vi "SVD demo.vi"(6 "number of points":i32(slide)=67 scale=0.0..600.0, 7 "gamma":dbl(slide) scale=-180.0..180.0, 8 "beta":dbl(slide) scale=-180.0..180.0, 9 "alpha":dbl(slide) scale=-180.0..180.0, 10 "length 2":dbl(slide)=5.0 scale=0.0..10.0, 11 "length 1":dbl(slide)=10.0 scale=0.0..10.0) -> ()   [LabVIEW 2009]
uses:
  <vilib>/Math Plots/3D Math Plots/3D Scatter/3D Scatter XCtrl/3D Scatter.xctl
  <vilib>/Math Plots/3D Math Plots/3D Scatter/3D Scatter Datatype/Public/Plot Helper (Vector).vi
  <vilib>/Analysis/Matrix/Numeric/Conversions/Matrix To Array - RM.vi
  <vilib>/Analysis/baseanly.llb/Real A x B.vi
  <vilib>/Analysis/Matrix/Numeric/Conversions/Array To Matrix - RA2.vi
  <vilib>/Analysis/Matrix/Numeric/Multiply/Multiply - RM,RM.vi
  <vilib>/Analysis/Matrix/NI_Matrix.lvlib
  <vilib>/Analysis/NI_AALBase.lvlib
  <vilib>/Math Plots/3D Math Plots/3D Scatter/3D Scatter Datatype/3D Scatter Datatype.lvclass
panel:
  out "Pre-Transformed data":refnum<class "3D Plot Datatype.lvclass">[](xcontrol)
  out "Transformed data":refnum<class "3D Plot Datatype.lvclass">[](xcontrol)
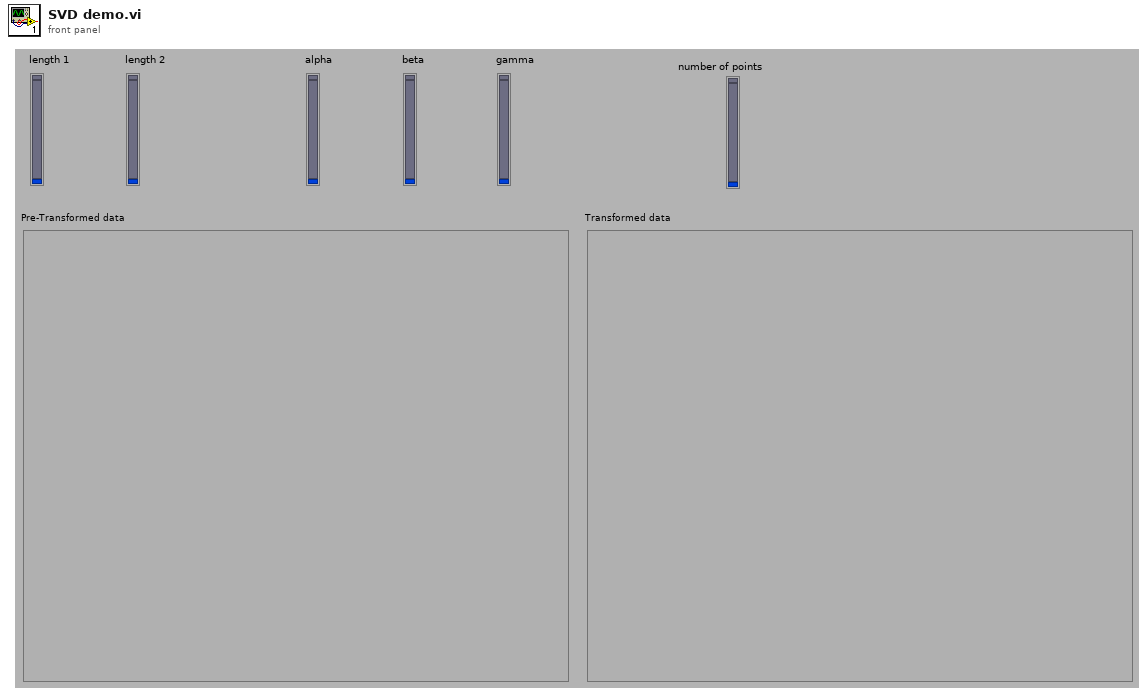
[diagram p1: front panel]
types:
  T1 = typedef "NI_Matrix.lvlib/RealMatrix.ctl" = dbl[][]
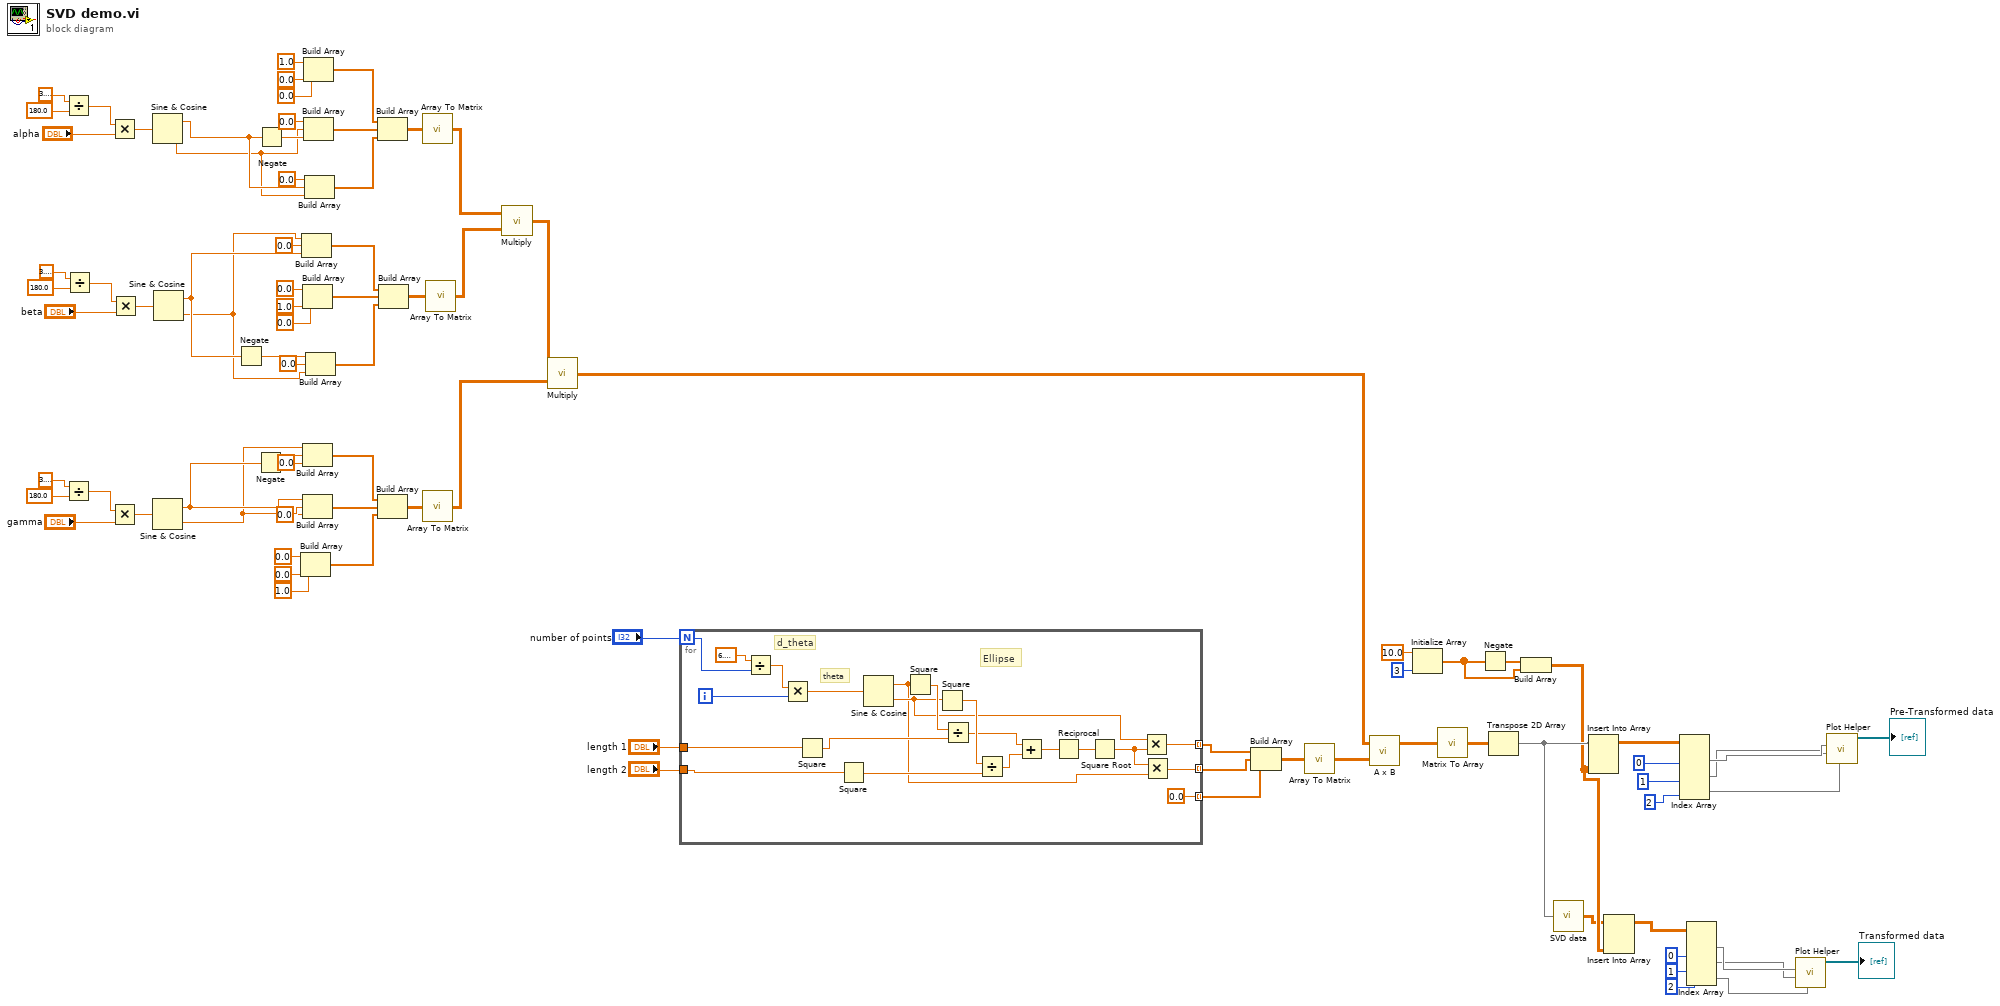
[diagram p0: block diagram]
diagram:
  n1 = Divide(x=3.141592653589793, y=180.0) -> (x/y=w84:dbl)
  n2 = Divide(x=3.141592653589793, y=180.0) -> (x/y=w69:dbl)
  n3 = Divide(x=3.141592653589793, y=180.0) -> (x/y=w62:dbl)
  n4 = Multiply(x=w84, y="alpha") -> (x*y=w83:dbl)
  n5 = Multiply(x=w69, y="gamma") -> (x*y=w68:dbl)
  n6 = Multiply(x=w62, y="beta") -> (x*y=w61:dbl)
  n7 = Sine & Cosine(0:w83) -> (1:w80:dbl, 2:w79:dbl)
  n8 = Sine & Cosine(0:w68) -> (1:w46:dbl, 2:w45:dbl)
  n9 = Sine & Cosine(0:w61) -> (1:w57:dbl, 2:w54:dbl)
  n10 = Negate(x=w57) -> (-x=w56:dbl)
  n11 = Negate(x=w46) -> (-x=w50:dbl)
  n12 = Negate(x=w80) -> (-x=w82:dbl)
  n13 = Build Array(0.0 ("element"), 0.0 ("element"), 1.0 ("element")) -> (w47:dbl[])
  n14 = Build Array(w54, 0.0 ("element"), w57) -> (w58:dbl[])
  n15 = Build Array(0.0 ("element"), 1.0 ("element"), 0.0 ("element")) -> (w59:dbl[])
  n16 = Build Array(w45, w50, 0.0 ("element")) -> (w48:dbl[])
  n17 = Build Array(w46, w45, 0.0 ("element")) -> (w43:dbl[])
  n18 = Build Array(1.0 ("element"), 0.0 ("element"), 0.0 ("element")) -> (w77:dbl[])
  n19 = Build Array(0.0 ("element"), w79, w82) -> (w76:dbl[])
  n20 = Build Array(0.0 ("element"), w80, w79) -> (w75:dbl[])
  n21 = Build Array(w56, 0.0 ("element"), w54) -> (w53:dbl[])
  n22 = Build Array(w77, w76, w75) -> (w42:dbl[][])
  n23 = Build Array(w48, w43, w47) -> (w40:dbl[][])
  n24 = Build Array(w58, w59, w53) -> (w41:dbl[][])
  n25 = call-poly <vilib>:"Array To Matrix.vi"("Real 2D Array"=w42) -> ("Real Matrix"=w39:T1)
  n26 = call-poly <vilib>:"Array To Matrix.vi"("Real 2D Array"=w40) -> ("Real Matrix"=w36:T1)
  n27 = call-poly <vilib>:"Array To Matrix.vi"("Real 2D Array"=w41) -> ("Real Matrix"=w38:T1)
  n28 = call-poly <vilib>:"Multiply.vi"("Real Matrix B"=w38, "Real Matrix A"=w39) -> ("A * B"=w37:T1)
  n29 = call-poly <vilib>:"Multiply.vi"("Real Matrix B"=w36, "Real Matrix A"=w37) -> ("A * B"=w27:T1)
  n30 = for {
    N: "number of points" -> [w109]
    tunnel: "length 1" -> [w101]
    tunnel: "length 2" -> [w99]
    tunnel: [w92] -> w32 mode=indexing
    tunnel: [w91] -> w31 mode=indexing
    tunnel: [0.0 ("y")] -> w29 mode=indexing
    i -> [w107]
    # "Ellipse"
    # "theta"
    # "d_theta"
    n31 = Divide(x=6.283185307179586, y=w109) -> (x/y=w108:dbl)
    n32 = Multiply(x=w108, y=w107) -> (x*y=w106:dbl)
    n33 = Square(x=w101) -> (x^2=w100:dbl)
    n34 = Square(x=w99) -> (x^2=w98:dbl)
    n35 = Sine & Cosine(0:w106) -> (1:w93:dbl, 2:w95:dbl)
    n36 = Square(x=w93) -> (x^2=w105:dbl)
    n37 = Square(x=w95) -> (x^2=w104:dbl)
    n38 = Divide(x=w105, y=w100) -> (x/y=w102:dbl)
    n39 = Divide(x=w104, y=w98) -> (x/y=w103:dbl)
    n40 = Add(x=w102, y=w103) -> (x+y=w97:dbl)
    n41 = Reciprocal(x=w97) -> (1/x=w96:dbl)
    n42 = Square Root(x=w96) -> (sqrt(x)=w94:dbl)
    n43 = Multiply(x=w95, y=w94) -> (x*y=w92:dbl)
    n44 = Multiply(x=w94, y=w93) -> (x*y=w91:dbl)
  }
  n45 = Build Array(w32, w31, w29) -> (w30:dbl[][])
  n46 = call-poly <vilib>:"Array To Matrix.vi"("Real 2D Array"=w30) -> ("Real Matrix"=w28:T1)
  n47 = call-poly <vilib>:"A x B.vi"("B"=w28, "A"=w27) -> ("A x B"=w26:T1)  [unwired: 1 out]
  n48 = Initialize Array(10.0 ("element"), 3 ("dimension size")) -> (w16:dbl[])
  n49 = call-poly <vilib>:"Matrix To Array.vi"("Real Matrix"=w26) -> ("Real 2D Array"=w20:dbl[][])
  n50 = Negate(x=w16) -> (-x=w15:dbl[])
  n51 = Transpose 2D Array(2D array=w20) -> (transposed array=w14:dbl[][])
  n52 = Build Array(w15, w16) -> (w12:dbl[][])
  n53 = call "SVD data.vi"("Data"=w14) -> ("Data out"=w11:dbl[][])
  n54 = Insert Into Array(array=w14, new element=w12) -> (w13:dbl[][])  [unwired: 2 in]
  n55 = Insert Into Array(array=w11, new element=w12) -> (w10:dbl[][])  [unwired: 2 in]
  n56 = Index Array(array=w13, index (col) #1=0 ("disabled index (col)"), index (col) #2=1 ("index (col)"), index (col) #3=2 ("index (col)")) -> (element #1=w7:dbl[], element #2=w6:dbl[], element #3=w5:dbl[])  [unwired: 3 in]
  n57 = Index Array(array=w10, index (col) #1=0 ("disabled index (col)"), index (col) #2=1 ("index (col)"), index (col) #3=2 ("index (col)")) -> (element #1=w4:dbl[], element #2=w3:dbl[], element #3=w2:dbl[])  [unwired: 3 in]
  n58 = call-poly <vilib>:"Plot Helper.vi"("z vector"=w2, "y vector"=w3, "x vector"=w4) -> ("3D Plot lvclass Array out"=→"Transformed data":refnum<class "3D Plot Datatype.lvclass">[])  [unwired: 3 in, 5 out]
  n59 = call-poly <vilib>:"Plot Helper.vi"("z vector"=w5, "y vector"=w6, "x vector"=w7) -> ("3D Plot lvclass Array out"=→"Pre-Transformed data":refnum<class "3D Plot Datatype.lvclass">[])  [unwired: 3 in, 5 out]
